vi "Test SMO Facade.vi"() -> ()   [LabVIEW 2013, in "SMOFacade.lvclass"]
uses:
  SMOFacade.lvclass
  SMO/SMO.lvclass
panel:
  out "error out 2":errorcluster
  out "Outputs":variant
  out "Public API":string[](array[string])
  out "method name":string
  out "error out":errorcluster
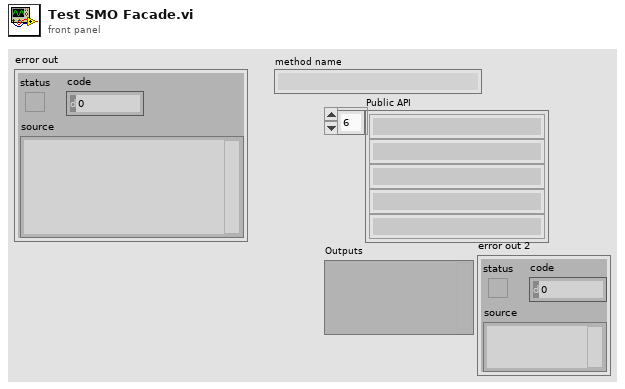
[diagram p1: front panel]
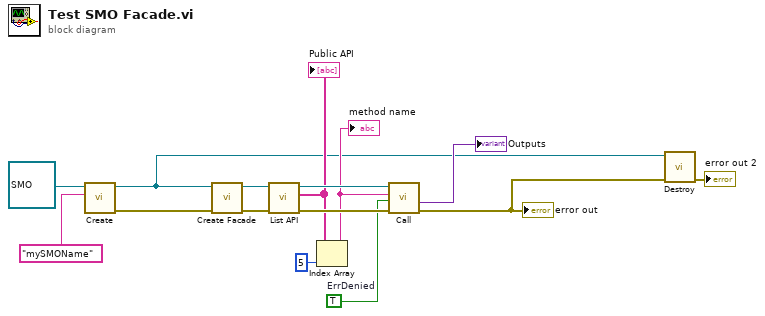
[diagram p0: block diagram]
diagram:
  w9 = TRUE  # ErrDenied
  n1 = call "Create.vi"("Subsystem Name (optional)"="mySMOName", "SMO"=refnum<class "SMO.lvclass"> refnum) -> ("error out"=w5:errorcluster, "SMO out"=w1:refnum<class "SMO.lvclass">)  [unwired: 7 in, 1 out]
  n2 = call "Create Facade.vi"("error in (no error)"=w5, "SMO"=w1) -> ("error out"=w14:errorcluster, "SMOFacade out"=w15:refnum<class "SMOFacade.lvclass">)  [unwired: 8 in]
  n3 = call "List API.vi"("error in (no error)"=w14, "SMOFacade in"=w15) -> ("error out"=w12:errorcluster, "Public API"=w8:string[], "SMOFacade out"=w13:refnum<class "SMOFacade.lvclass">)  [unwired: 7 in]
  "Public API" <- w8
  n4 = Index Array(array=w8, index=5) -> (element=w11:string)
  "method name" <- w11
  n5 = call "Call.vi"("error in (no error)"=w12, "Inputs"=w9, "Method Name"=w11, "SMOFacade in"=w13) -> ("error out"=w4:errorcluster, "Outputs"=→"Outputs":variant)  [unwired: 4 in, 2 out]
  "error out" <- w4
  n6 = call "Destroy.vi"("error in (no error)"=w4, "SMO"=w1) -> ("error out"=→"error out 2":errorcluster)  [unwired: 9 in]
